vi "REWORK_hex_whitespace_in_diagnostic_messages.vi"(11 "message_history":T1[](array[typedef])) -> (3 "hexed_records":string[][](array[string]))   [LabVIEW 2019]
uses:
  FGV/DIAGNOSTICS_message_history_buffer/REWORK_DIAGNOSTICS_message_history_buffer_all_info.ctl
  _misc/DIAGNOSTICS_message_type.ctl
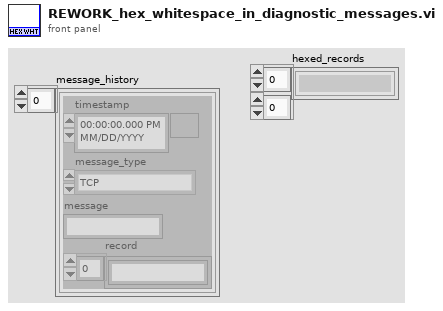
[diagram p1: front panel]
types:
  T1 = typedef "REWORK_DIAGNOSTICS_message_history_buffer_all_info.ctl" = cluster{"timestamp":timestamp, "message_type":T2, "message":string, "record":string[]}
  T2 = typedef "DIAGNOSTICS_message_type.ctl" = enum16{"TCP", "SQL"}
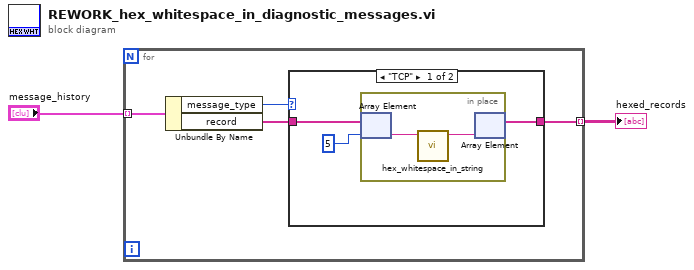
[diagram p0: block diagram]
diagram:
  n1 = for {
    tunnel: "message_history" -> [w6] mode=indexing
    tunnel: [w3] -> w2 mode=indexing
    n2 = Unbundle By Name(w6) -> ("message_type"=w5:T2, "record"=w4:string[])
    n3 = case shown="\"TCP\"" w5 {
      tunnel: w4 -> [w9 w12]
      tunnel: [w8 w12] -> w3
      frame "TCP" {
        n4 = in-place {
          n5 = in-place-array #1(w9, 5) -> (w11:string)
          n6 = call "hex_whitespace_in_string.vi"("string"=w11) -> ("hexed_string"=w10:string)  [unwired: 10 in]
          n7 = in-place-array #1(w10) -> (w8:string[])  [unwired: 1 out]
        }
      }
      frame "SQL" {
      }
    }
  }
  "hexed_records" <- w2
